vi "Write RM Addresses.vi"(6 "FIFO Idxs":i32[](array[numeric]), 8 "error in":errorcluster, 9 "Session":refnum<visa-resource-name>, 10 "Addresses":u32[](array[numeric]), 11 "Values":dbl[](array[numeric])) -> (0 "error out":errorcluster, 2 "Write Duration":u32, 3 "Values":dbl[](array[numeric]))   [LabVIEW 2019, in "GE_RM_Real Time.lvlib"]
uses:
  GE_RM_Real Time.lvlib
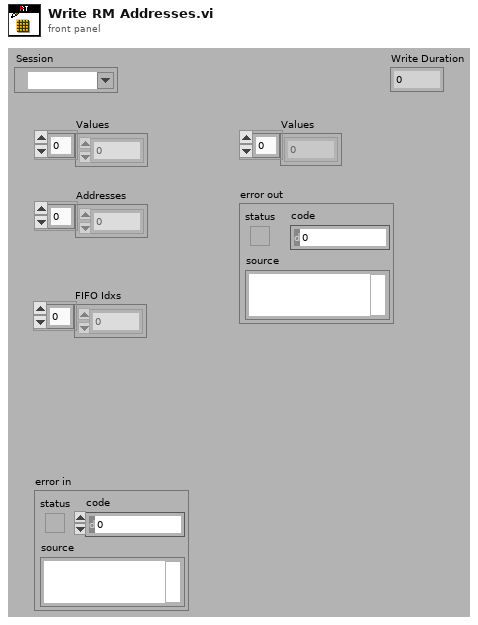
[diagram p1: front panel]
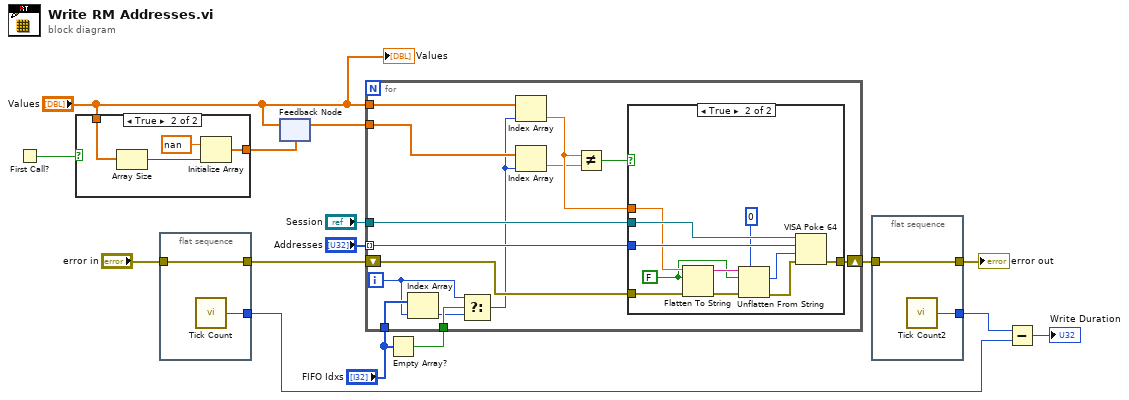
[diagram p0: block diagram]
diagram:
  n1 = First Call?() -> (First Call?: T/F=w4:bool)
  n2 = case shown="True" w4 {
    tunnel: "Values" -> [_ w19]
    tunnel: [_ w16] -> w2
    frame False {
    }
    frame True {
      n3 = Array Size(array=w19) -> (size(s)=w18:i32)
      n4 = Initialize Array(nan, w18) -> (w16:dbl[])
    }
  }
  n5 = flat-sequence {
    tunnel: [w21] -> w14
    tunnel: "error in" -> [w21]
    tunnel: [w20] -> w9
    frame #0 {
      n6 = call "Tick Count"() -> ("Tick Count(uSec)"=w20:u32)
    }
  }
  n7 = feedback-in #1("Values") -> ()
  n8 = feedback #1(w2) -> (w1:dbl[])
  n9 = Empty Array?(array="FIFO Idxs") -> (empty?=w6:bool)
  n10 = for "Write Output Values to System" {
    shift-right: [w33] -> w12
    shift-left: w14 -> [w27]
    tunnel: "Addresses" -> [w35] mode=indexing
    tunnel: "Session" -> [w34]
    tunnel: "Values" -> [w32]
    tunnel: w6 -> [w31]
    tunnel: "FIFO Idxs" -> [w30]
    tunnel: w1 -> [w26]
    i -> [w29]
    n11 = Index Array(array=w30, index=w29) -> (element=w28:i32)
    n12 = Select(t=w29, s=w31, f=w28) -> (s? t:f=w25:i32)
    n13 = Index Array(array=w32, index=w25) -> (element=w24:dbl)
    n14 = Index Array(array=w26, index=w25) -> (element=w23:dbl)
    n15 = Not Equal?(x=w24, y=w23) -> (x != y?=w22:bool)
    n16 = case shown="True" w22 {
      tunnel: w35 -> [_ w47]
      tunnel: w34 -> [_ w46]
      tunnel: [w36 w45] -> w33
      tunnel: w24 -> [_ w44]
      tunnel: w27 -> [w36 w38]
      frame False {
      }
      frame True {
        w37 = FALSE ("prepend array or string size? (T)")
        n17 = Flatten To String(anything=w44, prepend array or string size? (T)=w37, error in (no error)=w38) -> (data string=w42:string, error out=w43:errorcluster)  [unwired: 1 in, 1 out]
        n18 = Unflatten From String(type=u64 0 ("value (0)"), binary string=w42, data includes array or string size? (T)=w37, error in (no error)=w43) -> (value=w40:u64, error out=w39:errorcluster)  [unwired: 1 in, 1 out]
        n19 = VISA Poke 64(8:w39, 9:w40, 10:w47, 11:w46) -> (0:w45:errorcluster)  [unwired: 1 out]
      }
    }
  }
  n20 = flat-sequence {
    tunnel: [w49] -> w11
    tunnel: w12 -> [w49]
    tunnel: [w48] -> w10
    frame #0 {
      n21 = call "Tick Count2"() -> ("Tick Count(uSec)"=w48:u32)
    }
  }
  n22 = Subtract(x=w10, y=w9) -> (x-y=→"Write Duration":u32)
  "Values" <- "Values"
  "error out" <- w11
